vi "LoginPAI.vi"() -> ()   [LabVIEW 2024]
panel:
  in  "stop 2":bool
  in  "Tab Control":enum32{"Inicio", "Sistema"}(tab)
  in  "Open Button":bool
  in  "Contraseña":string
  in  "Usuario":string
  in  "Serie 2":bool
  in  "Serie 1":bool
  in  "stop":bool
  in  "COM":refnum<visa-resource-name>
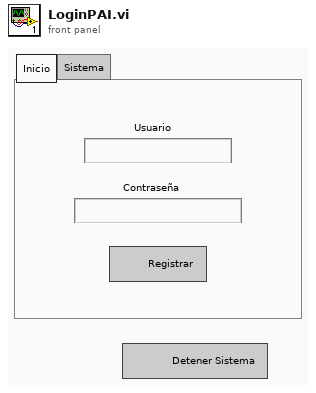
[diagram p1: front panel]
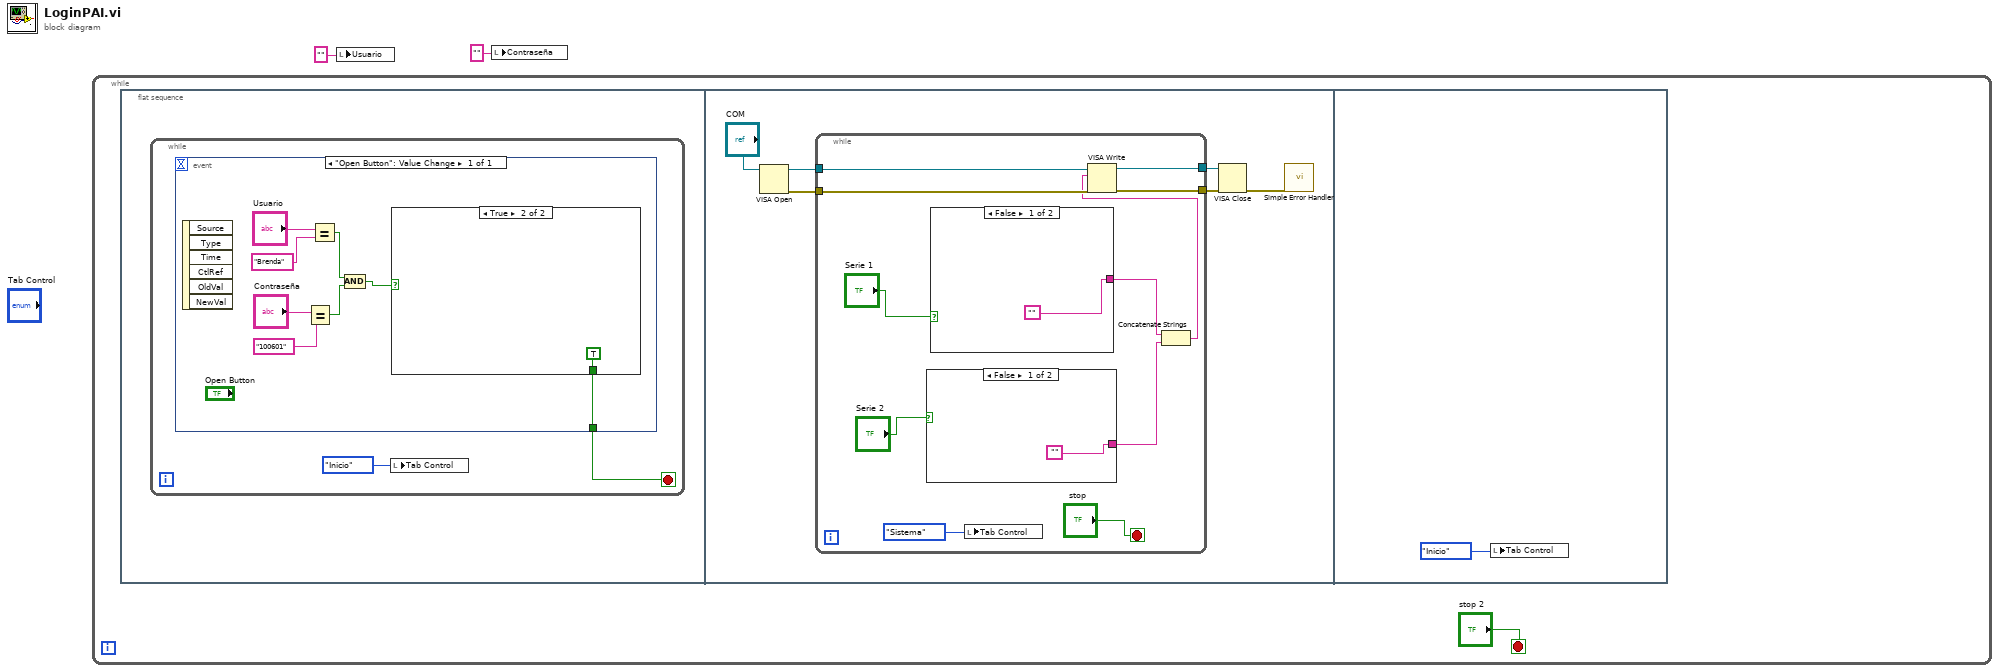
[diagram p0: block diagram]
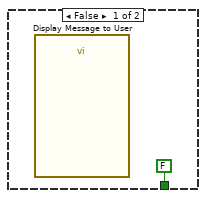
[diagram p2: hidden frame]
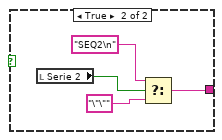
[diagram p3: hidden frame]
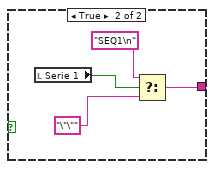
[diagram p4: hidden frame]
diagram:
  n1 = while {
    stop <- "stop 2" stop-if-true
    n2 = flat-sequence {
      frame #0 {
        n3 = while {
          stop <- w5 stop-if-true
          n4 = event shown="[0] \"Open Button\": Value Change" {
            selector: _ -> [_]
            dyn-events: _ -> [_]
            timeout: _ -> [_]
            tunnel: [w6] -> w5
            event "Open Button": Value Change {
              n5 = event-data() -> ()  [unwired: 1 in, 6 out]
              n6 = Equal?(x="Contraseña", y="100601") -> (x = y?=w8:bool)
              n7 = Equal?(x="Usuario", y="Brenda") -> (x = y?=w9:bool)
              n8 = And(x=w9, y=w8) -> (x .and. y?=w7:bool)
              n9 = case shown="True" w7 {
                tunnel: [FALSE TRUE] -> w6
                frame False {
                  n10 = call "Display Message to User"() -> ()  [unwired: 10 in, 2 out]
                }
                frame True {
                }
              }
            }
          }
          n11 = local write "Tab Control"(enum32{"Inicio", "Sistema"}."Inicio" ("Tab Control")) -> ()
        }
      }
      frame #1 {
        n12 = VISA Open(VISA resource name="COM") -> (VISA resource name=w21:refnum<visa-resource-name>, error out=w20:errorcluster)  [unwired: 4 in]
        n13 = while {
          tunnel: w21 -> [w31]
          tunnel: w20 -> [w30]
          tunnel: [w29] -> w17
          tunnel: [w28] -> w16
          stop <- "stop" stop-if-true
          n14 = case shown="False" "Serie 2" {
            tunnel: ["" w34] -> w24
            frame False {
            }
            frame True {
              n15 = local read "Serie 2"() -> (w37:bool)
              n16 = Select(t="SEQ2\n", s=w37, f="\"\"") -> (s? t:f=w34:string)
            }
          }
          n17 = case shown="False" "Serie 1" {
            tunnel: ["" w39] -> w26
            frame False {
            }
            frame True {
              n18 = local read "Serie 1"() -> (w40:bool)
              n19 = Select(t="SEQ1\n", s=w40, f="\"\"") -> (s? t:f=w39:string)
            }
          }
          n20 = local write "Tab Control"(enum32{"Inicio", "Sistema"}."Sistema" ("Tab Control")) -> ()
          n21 = Concatenate Strings(w26, w24) -> (w27:string)
          n22 = VISA Write(VISA resource name=w31, write buffer=w27, error in (no error)=w30) -> (VISA resource name out=w29:refnum<visa-resource-name>, error out=w28:errorcluster)  [unwired: 1 out]
        }
        n23 = VISA Close(VISA resource name=w17, error in (no error)=w16) -> (error out=w19:errorcluster)
        n24 = call <vilib>:"Simple Error Handler.vi"("error in (no error)"=w19) -> ()  [unwired: 4 in, 5 out]
      }
      frame #2 {
        n25 = local write "Tab Control"(enum32{"Inicio", "Sistema"}."Inicio" ("Tab Control")) -> ()
      }
    }
  }
  n26 = local write "Usuario"("" ("Usuario")) -> ()
  n27 = local write "Contraseña"("" ("Contraseña")) -> ()
